vi "eodrecorder_looping_open.vi"() -> ()   [LabVIEW 2012]
uses:
  eodrecorderstates.ctl
  <vilib>/Utility/error.llb/DialogType.ctl
  <vilib>/_DAQmxBase/Internals/DAQmxBase Create Channel (AI-Voltage-Basic).vi
  <vilib>/_DAQmxBase/Internals/DAQmxBase Timing (Sample Clock).vi
  <vilib>/_DAQmxBase/Internals/DAQmxBase Read (Analog 2D DBL NChan NSamp).vi
panel:
  out "Recording Length (sec.)":dbl
  in  "Threshold":sgl
  in  "NumSamptoGrab":i32
  in  "SampleRate":dbl=10000.0
  in  "Channel":tag="Dev1/ai0"
  out "String":string
  out "Tab Control":enum32{"Live Data", "Edit Data", "View Data"}(tab)
  in  "Discard&Continue":bool
  in  "Save&Finish":bool
  in  "Save&Continue":bool
  in  "StartOver":bool
  in  "Tab Control 2":enum32{"Enter Data", "View Data"}(tab)
  out "Time":string
  out "Date":string
  in  "Specimen No.":string
  in  "Locality Code":string
  in  "Recording Temp ûC":string
  in  "Comments":string
  in  "Species":string
  in  "Gain":dbl(knob) scale=0.0..10.0
  in  "Coupling":bool
  in  "Wave Number":u16(slide) scale=0.0..1.0
  out "WaveformDisplay":T1(array[cluster])
  out "EodText":string[](array[string])
  out "Polarity":i32[](array[numeric])
  out "Npts":i32[](array[numeric])
  out "Srate":i32[](array[numeric])
  out "ADRange":dbl[](array[numeric])
  in  "WaveNumber":i32(slide) max=4 scale=0.0..1.0
  out "Waveform Graph":dbl[][](graph) caption="Measurement"
  in  "LiveDataMode":bool
  in  "Capture":bool
  in  "Stop":bool
  in  "Open Data":bool
  # "EOD Recorder v. 0.1a"
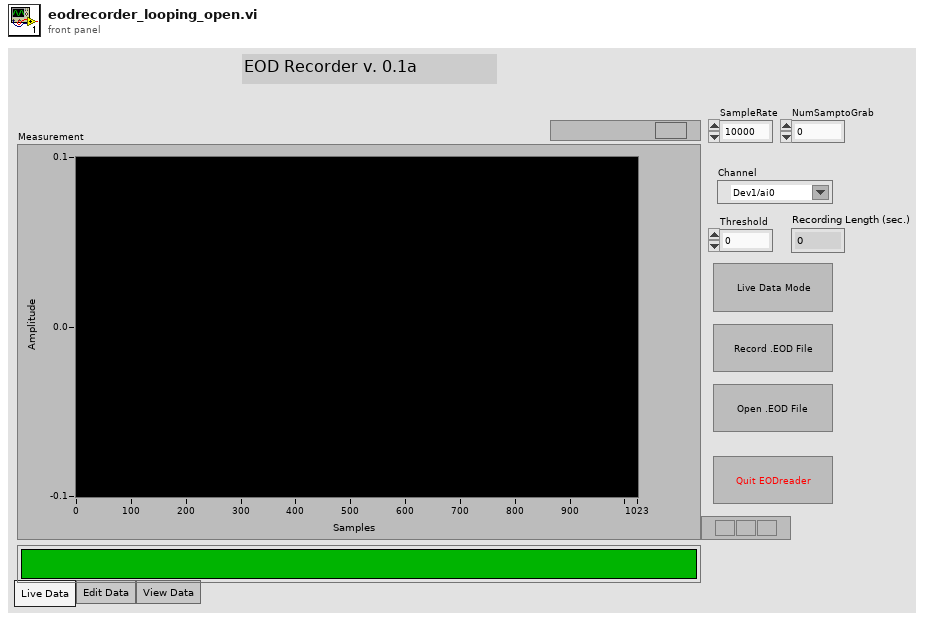
[diagram p1: front panel]
types:
  T1 = cluster{"Specimen No.":string, "Locality Code":string, "Species":string, "Recording Temp":string, "Comments 2":string, "Gain 2":dbl, "Coupling 2":bool, "Date 2":string, "Time 2":string}[]
  T2 = cluster{"data":dbl[][], "task ":refnum<k21>, "error ":errorcluster, "Min":dbl, "Max":dbl, "Srate":dbl, "WaveformData":cluster{"Nchar":i32[], "EodText":string[], "Nbits":i32[], "Nbytes":i32[], "userdata":dbl[][], "Polarity":i32[], "Srate":i32[], "ADRange":dbl[], "Npts":i32[], "Wave":dbl[][]}, "NumberofWavesLoaded":i32, "output array 2":cluster{"Specimen 2":string, "Location 2":string, "Species 2":string, "Temp 2":string, "Comments 2":string, "Gain 2":dbl, "Coupling 2":bool, "Date 2":string, "Time 2":string}[]}
  T3 = typedef "eodrecorderstates.ctl" = enum16{"stop", "initialize", "live data", "capture data", "analyze data", "open data", "display opened data", "write to file"}
  T4 = enum16{"Rising Edge", "Falling Edge", "Above Level", "Below Level", "When Inside Window", "When Outside Window"}
  T5 = enum16{"open", "replace", "create", "open or create", "replace or create", "replace or create with confirmation"}
  T6 = cluster{"Specimen 2":string, "Location 2":string, "Species 2":string, "Temp 2":string, "Comments 2":string, "Gain":dbl, "Coupling":bool, "Date 2":string, "Time 2":string}
  T7 = cluster{"Specimen 2":string, "Location 2":string, "Species 2":string, "Temp 2":string, "Comments 2":string, "Gain 2":dbl, "Coupling 2":bool, "Date 2":string, "Time 2":string}[]
  T8 = enum16{"big-endian, network order", "native, host order", "little-endian"}
  T9 = typedef "DialogType.ctl" = u16
  T10 = cluster{"Nchar":i32[], "EodText":string[], "Nbits":i32[], "Nbytes":i32[], "userdata":dbl[][], "Polarity":i32[], "Srate":i32[], "ADRange":dbl[], "Npts":i32[], "Wave":dbl[][]}
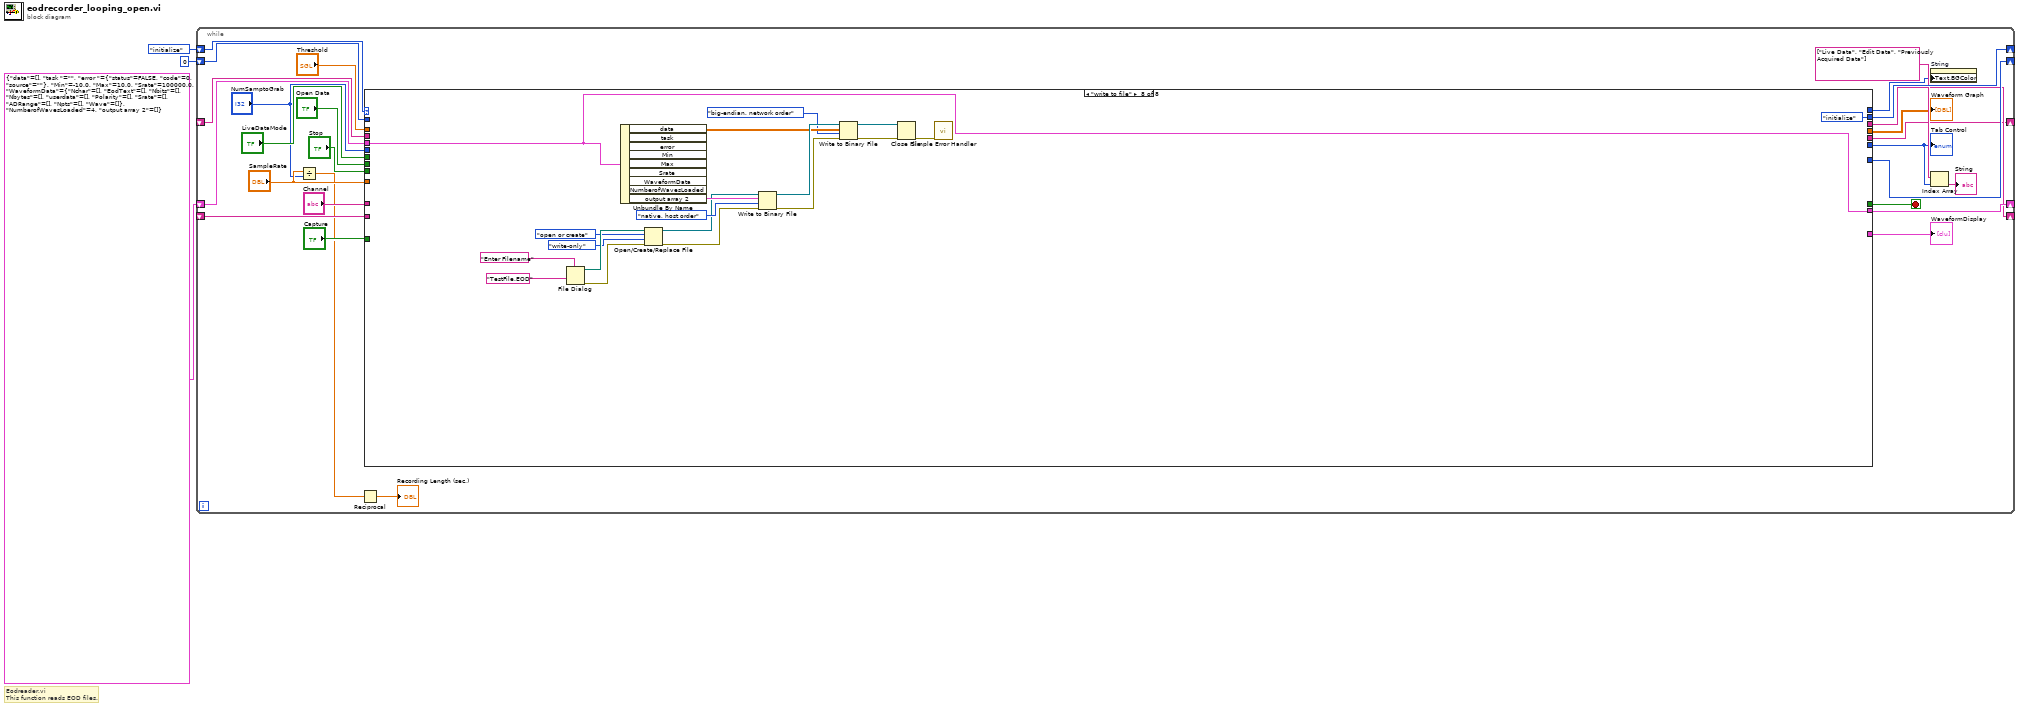
[diagram p0: block diagram]
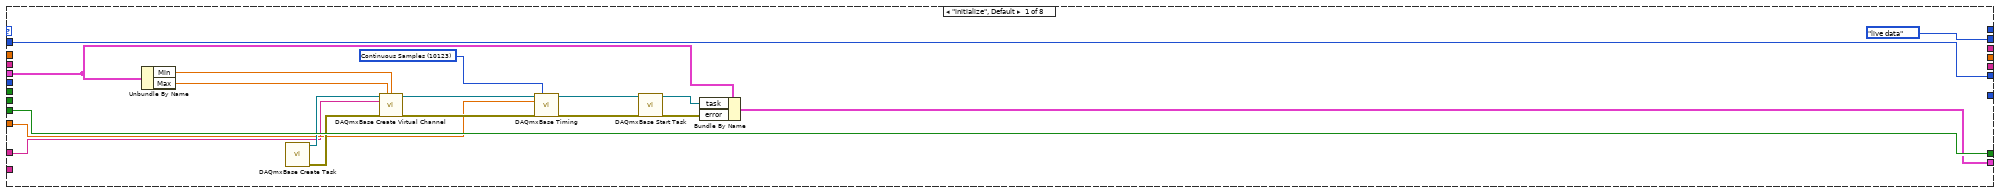
[diagram p2: hidden frame]
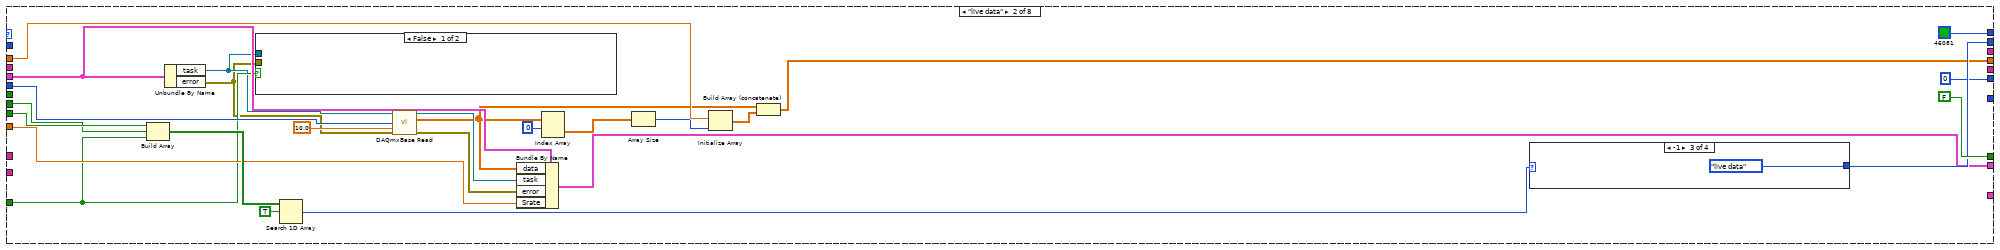
[diagram p3: hidden frame]
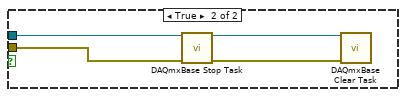
[diagram p4: hidden frame]
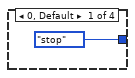
[diagram p5: hidden frame]
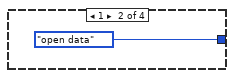
[diagram p6: hidden frame]
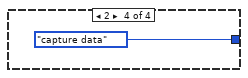
[diagram p7: hidden frame]
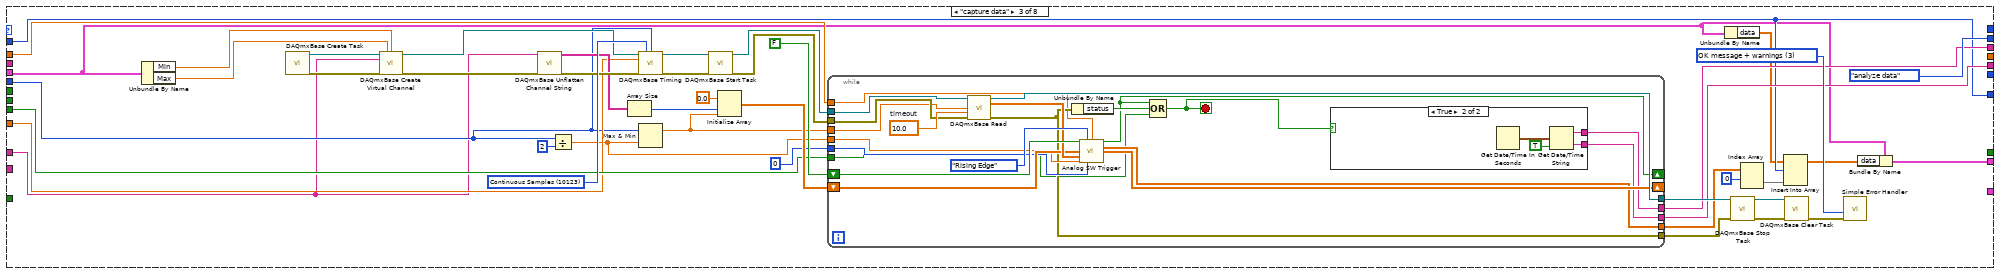
[diagram p8: hidden frame]
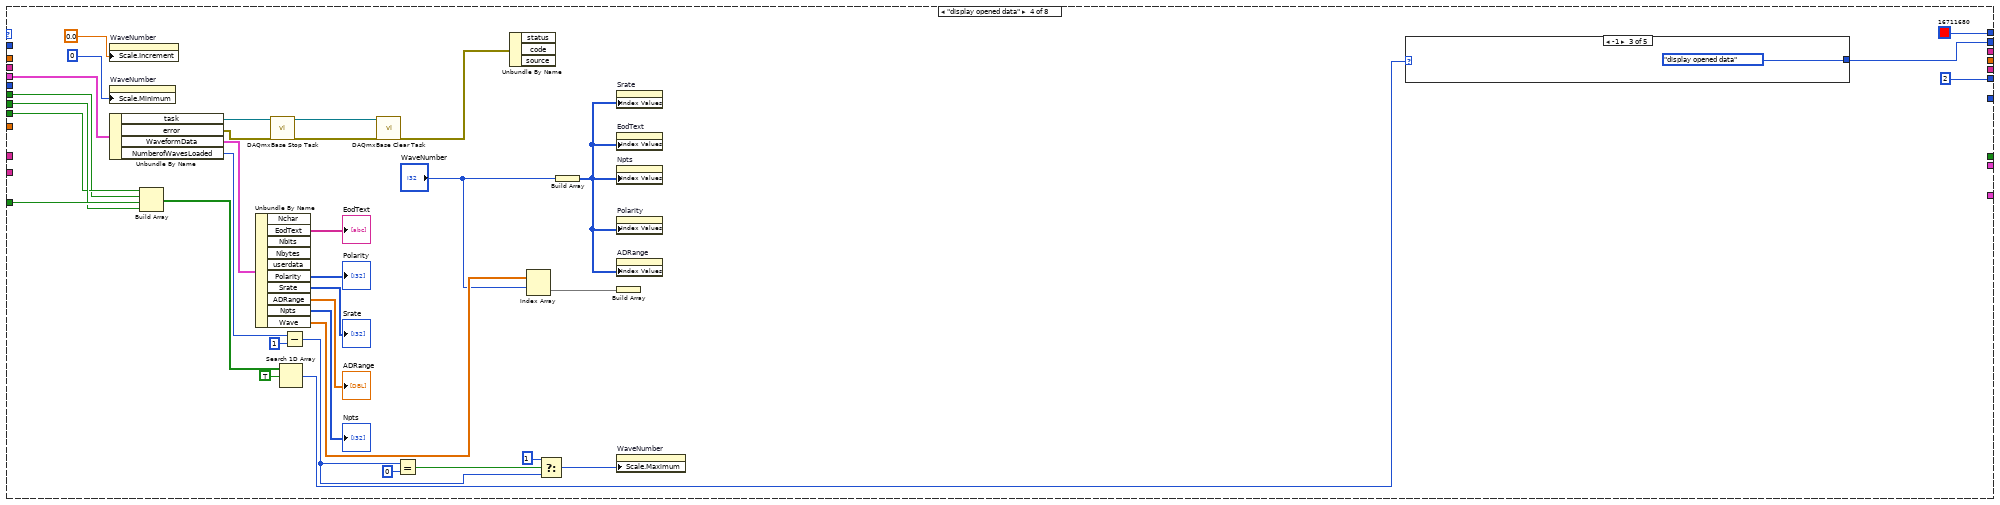
[diagram p10: hidden frame]
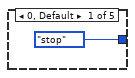
[diagram p11: hidden frame]
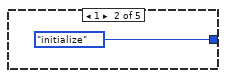
[diagram p12: hidden frame]
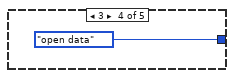
[diagram p13: hidden frame]
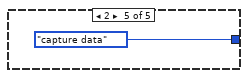
[diagram p14: hidden frame]
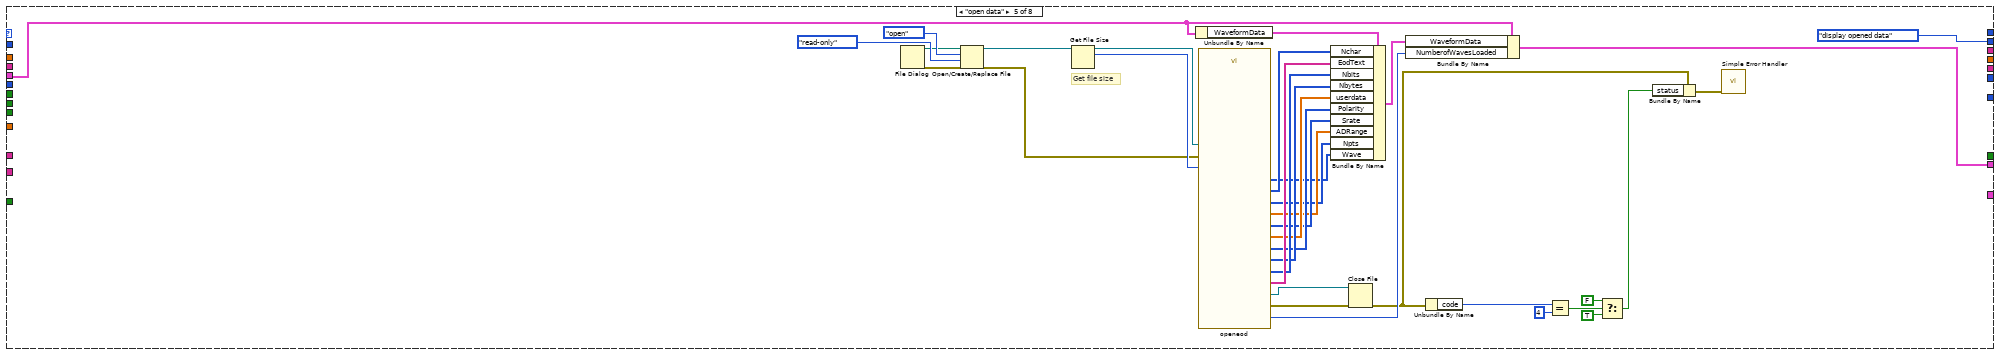
[diagram p15: hidden frame]
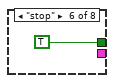
[diagram p16: hidden frame]
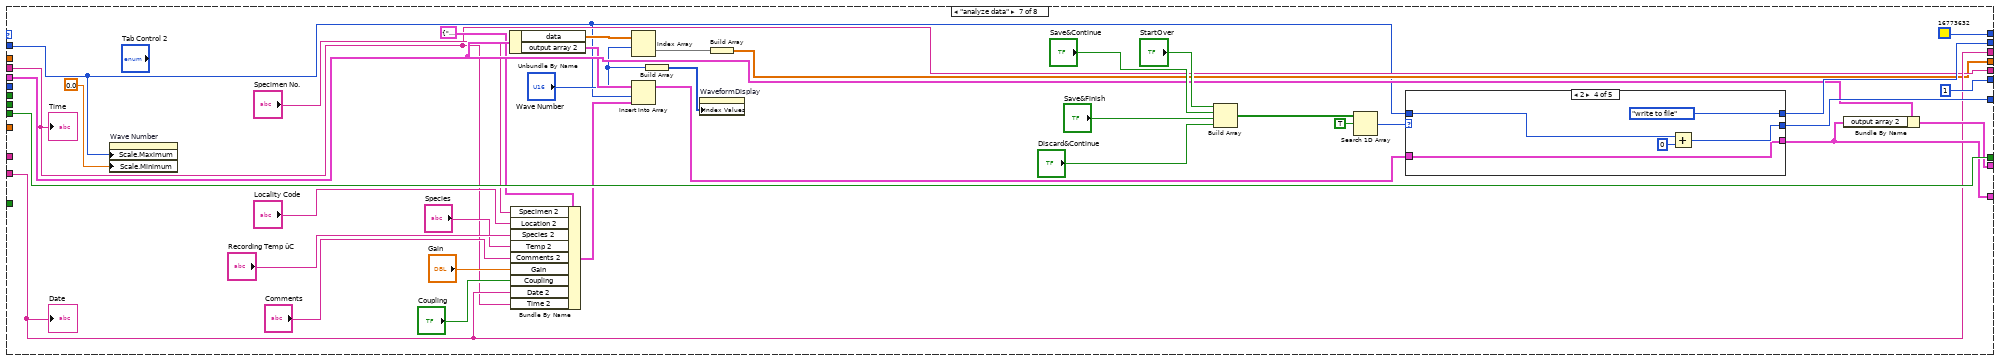
[diagram p17: hidden frame]
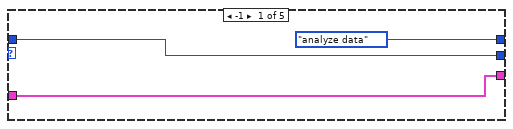
[diagram p18: hidden frame]
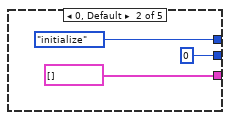
[diagram p19: hidden frame]
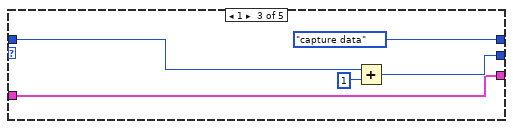
[diagram p20: hidden frame]
diagram:
  # "Eodreader.vi\nThis function reads EOD files."
  n1 = while {
    shift-right: [w29] -> _
    shift-left: eodrecorderstates."initialize" ("Enum") -> [w22]
    shift-right: [w15] -> _
    shift-left: T2 {"data"=[], "task "="", "error "={"status"=FALSE, "code"=0, "source"=""}, "Min"=-10.0, "Max"=10.0, "Srate"=100000.0, "WaveformData"={"Nchar"=[], "EodText"=[], "Nbits"=[], "Nbytes"=[], "userdata"=[], "Polarity"=[], "Srate"=[], "ADRange"=[], "Npts"=[], "Wave"=[]}, "NumberofWavesLoaded"=4, "output array 2"=[]} -> [w27]
    shift-right: [w16] -> _
    shift-left: u16 0 -> [w17]
    shift-right: [w12] -> _
    shift-left: _ -> [w10]
    shift-right: [w11] -> _
    shift-left: _ -> [w9]
    stop <- w30 stop-if-true
    n2 = Divide(x="SampleRate", y="NumSamptoGrab") -> (x/y=w5:dbl)
    n3 = Reciprocal(x=w5) -> (1/x=→"Recording Length (sec.)":dbl)
    n4 = case shown="\"write to file\"" w22 {
      tunnel: [w47 FALSE _ _ _ TRUE w257 _] -> w30
      tunnel: [eodrecorderstates."live data" ("Enum") w73 eodrecorderstates."analyze data" ("Enum") w185 eodrecorderstates."display opened data" ("Enum") _ w256 eodrecorderstates."initialize" ("Enum")] -> w29
      tunnel: "Stop" -> [w47 w72 w100 w179 _ _ w257 _]
      tunnel: w27 -> [w34 w68 w85 w151 w193 _ w247 w282]
      tunnel: "NumSamptoGrab" -> [_ w64 w97 _ _ _ _ _]
      tunnel: "SampleRate" -> [w35 w62 w98 _ _ _ _ _]
      tunnel: "Open Data" -> [_ w63 _ w181 _ _ _ _]
      tunnel: "Capture" -> [_ w60 _ w182 _ _ _ _]
      tunnel: "LiveDataMode" -> [_ _ _ w178 _ _ _ _]
      tunnel: "Threshold" -> [_ w61 w99 _ _ _ _ _]
      tunnel: [w33 0 _ 2 _ _ 1 _] -> w19
      tunnel: [_ u32 46081 _ u32 16711680 _ _ u32 16773632 _] -> w18
      tunnel: w17 -> [w33 _ w87 _ _ _ w226 _]
      tunnel: [_ _ w87 _ _ _ w255 _] -> w16
      tunnel: [w31 w50 w92 _ w191 _ w246 w282] -> w15
      tunnel: "Channel" -> [w32 _ w93 _ _ _ _ _]
      tunnel: [_ _ _ _ _ _ w244 _] -> w13
      tunnel: [_ _ w91 _ _ _ w234 _] -> w12
      tunnel: [_ _ w90 _ _ _ w233 _] -> w11
      tunnel: w10 -> [_ _ _ _ _ _ w234 _]
      tunnel: w9 -> [_ _ _ _ _ _ w233 _]
      tunnel: [_ w49 _ _ _ _ w228 _] -> w8
      frame "initialize", Default {
        w42 = 10123 items=["Finite Samples"=10178, "Continuous Samples"=10123] ("sample mode")
        n5 = Unbundle By Name(w34) -> ("Min"=w39:dbl, "Max"=w38:dbl)
        n6 = call <vilib>:"DAQmxBase Create Task.vi"() -> ("task out"=w45:refnum<k21>, "error out"=w46:errorcluster)  [unwired: 5 in, 9 out]
        n7 = call-poly <vilib>:"DAQmxBase Create Virtual Channel.vi"("task in"=w45, "maximum value"=w38, "minimum value"=w39, "physical channels"=w32, "error in"=w46) -> ("task out"=w43:refnum<k21>, "error out"=w44:errorcluster)  [unwired: 4 in, 5 out]
        n8 = call-poly <vilib>:"DAQmxBase Timing.vi"("task/channels in"=w43, "sample mode"=w42, "rate"=w35, "error in"=w44) -> ("task out"=w37:refnum<k21>, "error out"=w36:errorcluster)  [unwired: 3 in, 7 out]
        n9 = call <vilib>:"DAQmxBase Start Task.vi"("task/channels in"=w37, "error in"=w36) -> ("task out"=w41:refnum<k21>, "error out"=w40:errorcluster)  [unwired: 12 out]
        n10 = Bundle By Name(cluster=w34, "task"=w41, "error"=w40) -> (w31:T2)
      }
      frame "live data" {
        n11 = Build Array(w72, w63, w60) -> (w71:bool[])
        n12 = Unbundle By Name(w68) -> ("task"=w59:refnum<k21>, "error"=w58:errorcluster)
        n13 = case shown="False" w60 {
          tunnel: w59 -> [_ w78]
          tunnel: w58 -> [_ w77]
          frame False {
          }
          frame True {
            n14 = call <vilib>:"DAQmxBase Stop Task.vi"("task/channels in"=w78, "error in"=w77) -> ("task out"=w76:refnum<k21>, "error out"=w75:errorcluster)  [unwired: 12 in]
            n15 = call <vilib>:"DAQmxBase Clear Task.vi"("task in"=w76, "error in"=w75) -> ()  [unwired: 13 in, 1 out]
          }
        }
        n16 = Search 1D Array(1D array=w71, element=TRUE) -> (index of element=w69:i32)  [unwired: 1 in]
        n17 = call-poly <vilib>:"DAQmxBase Read.vi"("task/channels in"=w59, "number of samples per channel"=w64, "timeout"=10.0, "error in"=w58) -> ("task out"=w67:refnum<k21>, "data"=w53:dbl[][], "error out"=w66:errorcluster)  [unwired: 9 out]
        n18 = Bundle By Name(cluster=w68, "data"=w53, "task"=w67, "error"=w66, "Srate"=w62) -> (w50:T2)
        n19 = Index Array(array=w53, index (row)=0) -> (element=w55:dbl[])  [unwired: 1 in]
        n20 = Array Size(array=w55) -> (size(s)=w56:i32)
        n21 = Initialize Array(w61, w56) -> (w54:sgl[])
        n22 = Build Array (concatenate)(w53, w54) -> (w49:dbl[][])
        n23 = case shown="-1" w69 {
          tunnel: [eodrecorderstates."stop" ("Enum") eodrecorderstates."open data" ("Enum") eodrecorderstates."live data" ("Enum") eodrecorderstates."capture data" ("Enum")] -> w73
          frame 0, Default {
          }
          frame 1 {
          }
          frame -1 {
          }
          frame 2 {
          }
        }
      }
      frame "capture data" {
        w105 = T9 3 items=["no dialog", "OK message", "continue or stop message", "OK message + warnings", "continue/stop + warnings"] ("type of dialog (OK msg:1)")
        w125 = 10123 items=["Finite Samples"=10178, "Continuous Samples"=10123] ("sample mode")
        n24 = Unbundle By Name(w85) -> ("Min"=w122:dbl, "Max"=w121:dbl)
        n25 = call <vilib>:"DAQmxBase Create Task.vi"() -> ("task out"=w124:refnum<k21>, "error out"=w123:errorcluster)  [unwired: 14 in]
        n26 = call-poly <vilib>:"DAQmxBase Create Virtual Channel.vi"("task in"=w124, "maximum value"=w121, "minimum value"=w122, "physical channels"=w93, "error in"=w123) -> ("task out"=w120:refnum<k21>, "error out"=w117:errorcluster)  [unwired: 9 in]
        n27 = call "DAQmxBase Unflatten Channel String.vi"("names in"=w93, "error in"=w117) -> ("names out"=w115:string[], "error out"=w116:errorcluster)  [unwired: 12 in]
        n28 = Divide(x=w97, y=2) -> (x/y=w95:dbl)
        n29 = Array Size(array=w115) -> (size(s)=w114:i32)
        n30 = call-poly <vilib>:"DAQmxBase Timing.vi"("task/channels in"=w120, "sample mode"=w125, "samples per channel"=w97, "rate"=w98, "error in"=w116) -> ("task out"=w119:refnum<k21>, "error out"=w118:errorcluster)  [unwired: 2 in, 7 out]
        n31 = Max & Min(x=w97, y=w95) -> (max(x,y)=w107:dbl)  [unwired: 1 out]
        n32 = call <vilib>:"DAQmxBase Start Task.vi"("task/channels in"=w119, "error in"=w118) -> ("task out"=w111:refnum<k21>, "error out"=w112:errorcluster)  [unwired: 12 out]
        n33 = Initialize Array(0.0, w114, w107) -> (w110:dbl[][])
        n34 = while {
          tunnel: [w140] -> w102
          shift-right: [w139] -> _
          shift-left: FALSE ("Trigger Out") -> [w145]
          shift-right: [w133] -> _
          shift-left: w110 -> [w141]
          tunnel: w112 -> [w138]
          tunnel: w111 -> [w137]
          tunnel: w95 -> [w136]
          tunnel: 0 ("Channel Index") -> [w135]
          tunnel: w107 -> [w134]
          tunnel: [w132] -> w89
          tunnel: [w131] -> w101
          tunnel: w100 -> [w130]
          tunnel: w99 -> [w129]
          tunnel: [w127] -> w91
          tunnel: [w126] -> w90
          stop <- w128 stop-if-true
          w146 = 10.0  # timeout
          n35 = call-poly <vilib>:"DAQmxBase Read.vi"("task/channels in"=w137, "number of samples per channel"=w134, "timeout"=w146, "error in"=w138) -> ("task out"=w140:refnum<k21>, "data"=w142:dbl[][], "error out"=w131:errorcluster)  [unwired: 9 in]
          n36 = Unbundle By Name(w131) -> ("status"=w144:bool)
          n37 = call "Analog SW Trigger.vi"("Triggered?"=w145, "Condition"=T4."Rising Edge", "Level"=w129, "Initialized Data Array"=w141, "Input Raw Data"=w142, "Pretrigger Samples"=w136, "Index of Condition Channel"=w135) -> ("Trigger Out"=w139:bool, "Output Data (Scaled)"=w132:dbl[][], "Raw Data Out"=w133:dbl[][])  [unwired: 4 in, 2 out]
          n38 = Compound Arithmetic op=OR(w139, w144, w130) -> (w128:bool)
          n39 = case shown="True" w128 {
            tunnel: [_ w148] -> w127
            tunnel: [_ w147] -> w126
            frame False {
            }
            frame True {
              n40 = Get Date/Time In Seconds() -> (seconds since 1Jan1904=w150:timestamp)
              n41 = Get Date/Time String(seconds (now)=w150, want seconds? (F)=TRUE) -> (date string=w148:string, time string=w147:string)  [unwired: 1 in]
            }
          }
        }
        n42 = Unbundle By Name(w85) -> ("data"=w84:dbl[][])
        n43 = call <vilib>:"DAQmxBase Stop Task.vi"("task/channels in"=w102, "error in"=w101) -> ("task out"=w104:refnum<k21>, "error out"=w103:errorcluster)  [unwired: 12 in]
        n44 = Index Array(array=w89, index (row)=0) -> (element=w83:dbl[])  [unwired: 1 in]
        n45 = Insert Into Array(array=w84, index (row)=w87, new element=w83) -> (w86:dbl[][])  [unwired: 1 in]
        n46 = call <vilib>:"DAQmxBase Clear Task.vi"("task in"=w104, "error in"=w103) -> ("error out"=w106:errorcluster)  [unwired: 13 in]
        n47 = call <vilib>:"Simple Error Handler.vi"("type of dialog (OK msg:1)"=w105, "error in (no error)"=w106) -> ()  [unwired: 3 in, 5 out]
        n48 = Bundle By Name(cluster=w85, "data"=w86) -> (w92:T2)
      }
      frame "display opened data" {
        n49 = property on="WaveNumber" class="Slide (strict)"("Scale.Increment"=0.0 ("Scale.Range:Increment")) -> ()  [unwired: 2 in, 2 out]
        n50 = property on="WaveNumber" class="Slide (strict)"("Scale.Minimum"=0) -> ()  [unwired: 2 in, 2 out]
        n51 = Unbundle By Name(w151) -> ("task"=w174:refnum<k21>, "error"=w173:errorcluster, "WaveformData"=w172:T10, "NumberofWavesLoaded"=w160:i32)
        n52 = Build Array(w179, w178, w182, w181) -> (w184:bool[])
        n53 = Unbundle By Name(w172) -> ("EodText"=→"EodText":string[], "Polarity"=→"Polarity":i32[], "Srate"=→"Srate":i32[], "ADRange"=→"ADRange":dbl[], "Npts"=→"Npts":i32[], "Wave"=w164:dbl[][])  [unwired: 4 out]
        n54 = call <vilib>:"DAQmxBase Stop Task.vi"("task/channels in"=w174, "error in"=w173) -> ("task out"=w175:refnum<k21>, "error out"=w176:errorcluster)  [unwired: 12 in]
        n55 = Search 1D Array(1D array=w184, element=TRUE) -> (index of element=w180:i32)  [unwired: 1 in]
        n56 = Subtract(x=w160, y=1) -> (x-y=w155:i32)
        n57 = call <vilib>:"DAQmxBase Clear Task.vi"("task in"=w175, "error in"=w176) -> ("error out"=w177:errorcluster)  [unwired: 13 in]
        n58 = Equal?(x=w155, y=0) -> (x = y?=w156:bool)
        n59 = Unbundle By Name(w177) -> ()  [unwired: 3 out]
        n60 = Index Array(array=w164, index (row)="WaveNumber") -> (element=w162:dbl[])  [unwired: 1 in]
        n61 = Select(t=1, s=w156, f=w155) -> (s? t:f=w153:i32)
        n62 = Build Array("WaveNumber") -> (w166:i32[])
        n63 = property on="Srate" class="Arr (strict)"("Index Values"=w166) -> ()  [unwired: 2 in, 2 out]
        n64 = property on="EodText" class="Arr (strict)"("Index Values"=w166) -> ()  [unwired: 2 in, 2 out]
        n65 = property on="Npts" class="Arr (strict)"("Index Values"=w166) -> ()  [unwired: 2 in, 2 out]
        n66 = property on="Polarity" class="Arr (strict)"("Index Values"=w166) -> ()  [unwired: 2 in, 2 out]
        n67 = property on="ADRange" class="Arr (strict)"("Index Values"=w166) -> ()  [unwired: 2 in, 2 out]
        n68 = Build Array(w162) -> ()  [unwired: 1 out]
        n69 = property on="WaveNumber" class="Slide (strict)"("Scale.Maximum"=w153) -> ()  [unwired: 2 in, 2 out]
        n70 = case shown="-1" w180 {
          tunnel: [eodrecorderstates."stop" ("Enum") eodrecorderstates."initialize" ("Enum") eodrecorderstates."display opened data" ("Enum") eodrecorderstates."open data" ("Enum") eodrecorderstates."capture data" ("Enum")] -> w185
          frame 0, Default {
          }
          frame 1 {
          }
          frame -1 {
          }
          frame 3 {
          }
          frame 2 {
          }
        }
      }
      frame "open data" {
        # "Get file size"
        n71 = File Dialog() -> (0:w220:errorcluster, 3:w221:path)  [unwired: 7 in, 2 out]
        n72 = Open/Create/Replace File(file path (use dialog)=w221, error in=w220, operation (0:open)=T5."open", access (0:read/write)=enum16{"read/write", "read-only", "write-only"}."read-only") -> (refnum out=w209:refnum<file>, error out=w202:errorcluster)  [unwired: 2 in, 1 out]
        n73 = Get File Size(file=w209) -> (refnum out=w208:refnum<file>, size (in bytes)=w207:i64)  [unwired: 1 in, 1 out]
        n74 = Unbundle By Name(w193) -> ("WaveformData"=w219:T10)
        n75 = call "openeod.vi"("Byte Stream File in"=w208, "size (in bytes)"=w207, "error in (no error)"=w202) -> ("Wave"=w192:i16[][], "nchar"=w218:u8[], "polarity"=w214:i8[], "nWavepoints"=w210:u32[], "userdata"=w213:sgl[][], "Numeric"=w205:i32, "nbytes"=w215:i8[], "Byte Stream File out"=w204:refnum<file>, "ADrange"=w211:sgl[], "eodtext"=w217:string[], "srate"=w212:u32[], "nbits"=w216:i8[], "error out"=w203:errorcluster)  [unwired: 4 in]
        n76 = Bundle By Name(cluster=w219, "Nchar"=w218, "EodText"=w217, "Nbits"=w216, "Nbytes"=w215, "userdata"=w213, "Polarity"=w214, "Srate"=w212, "ADRange"=w211, "Npts"=w210, "Wave"=w192) -> (w206:T10)
        n77 = Close File(refnum=w204, error in=w203) -> (error out=w194:errorcluster)  [unwired: 1 out]
        n78 = Bundle By Name(cluster=w193, "WaveformData"=w206, "NumberofWavesLoaded"=w205) -> (w191:T2)
        n79 = Unbundle By Name(w194) -> ("code"=w201:i32)
        n80 = Equal?(x=w201, y=4) -> (x = y?=w199:bool)
        n81 = Select(t=FALSE, s=w199, f=TRUE) -> (s? t:f=w196:bool)
        n82 = Bundle By Name(cluster=w194, "status"=w196) -> (w195:errorcluster)
        n83 = call <vilib>:"Simple Error Handler.vi"("error in (no error)"=w195) -> ()  [unwired: 4 in, 5 out]
      }
      frame "stop" {
      }
      frame "analyze data" {
        n84 = property on="Wave Number" class="Slide (strict)"("Scale.Maximum"=w226, "Scale.Minimum"=0.0 ("Scale.Range:Minimum")) -> ()  [unwired: 2 in, 2 out]
        n85 = Unbundle By Name(w247) -> ("data"=w232:dbl[][], "output array 2"=w245:T7)
        n86 = Bundle By Name(cluster=T6 {"Specimen 2"="", "Location 2"="", "Species 2"="", "Temp 2"="", "Comments 2"="", "Gain"=50.0, "Coupling"=TRUE, "Date 2"="", "Time 2"=""} ("WaveformDescribe 2"), "Specimen 2"="Specimen No.", "Location 2"="Locality Code", "Species 2"="Species", "Temp 2"="Recording Temp ûC", "Comments 2"="Comments", "Gain"="Gain", "Coupling"="Coupling", "Date 2"=w234, "Time 2"=w233) -> (w235:T6)
        n87 = Index Array(array=w232, index (row)="Wave Number") -> (element=w229:dbl[])  [unwired: 1 in]
        n88 = Insert Into Array(array=w245, index=w226, new element=w235) -> (w249:T7)
        n89 = Build Array("Wave Number") -> (w231:u16[])
        n90 = property on="WaveformDisplay" class="Arr (strict)"("Index Values"=w231) -> ()  [unwired: 2 in, 2 out]
        n91 = Build Array(w229) -> (w228:dbl[][])
        n92 = Build Array("StartOver", "Save&Continue", "Save&Finish", "Discard&Continue") -> (w258:bool[])
        n93 = Search 1D Array(1D array=w258, element=TRUE) -> (index of element=w250:i32)  [unwired: 1 in]
        n94 = case shown="2" w250 {
          tunnel: [w262 0 w270 w275 w280] -> w255
          tunnel: w226 -> [w262 _ w269 w274 w279]
          tunnel: [eodrecorderstates."analyze data" ("Enum") eodrecorderstates."initialize" ("Enum") eodrecorderstates."capture data" ("Enum") eodrecorderstates."write to file" ("Enum") eodrecorderstates."capture data" ("Enum")] -> w256
          tunnel: [w261 T7 [] ("output array 2") w267 w272 w277] -> w244
          tunnel: w249 -> [w261 _ w267 w272 w277]
          frame -1 {
          }
          frame 0, Default {
          }
          frame 1 {
            n95 = Add(x=w269, y=1) -> (x+y=w270:i32)
          }
          frame 2 {
            n96 = Add(x=w274, y=0) -> (x+y=w275:i32)
          }
          frame 3 {
            n97 = Add(x=w279, y=0) -> (x+y=w280:i32)
          }
        }
        n98 = Bundle By Name(cluster=w247, "output array 2"=w244) -> (w246:T2)
        "Time" <- w233
        "Date" <- w234
      }
      frame "write to file" {
        n99 = File Dialog(7:"Enter Filename" ("prompt"), 9:"TestFile.EOD" ("default name")) -> (0:w292:errorcluster, 3:w298:path)  [unwired: 5 in, 2 out]
        n100 = Unbundle By Name(w282) -> ("data"=w285:dbl[][], "output array 2"=w300:T7)  [unwired: 7 out]
        n101 = Open/Create/Replace File(file path (use dialog)=w298, error in=w292, operation (0:open)=T5."open or create", access (0:read/write)=enum16{"read/write", "read-only", "write-only"}."write-only") -> (refnum out=w294:refnum<file>, error out=w293:errorcluster)  [unwired: 2 in, 1 out]
        n102 = Write to Binary File(file (use dialog)=w294, data=w300, error in=w293, 9:T8."native, host order" ("byte order (0:big-endian, network order)")) -> (refnum out=w289:refnum<file>, error out=w288:errorcluster)  [unwired: 2 in, 1 out]
        n103 = Write to Binary File(file (use dialog)=w289, data=w285, error in=w288, 9:T8."big-endian, network order" ("byte order (0:big-endian, network order)")) -> (refnum out=w286:refnum<file>, error out=w287:errorcluster)  [unwired: 2 in, 1 out]
        n104 = Close File(refnum=w286, error in=w287) -> (error out=w291:errorcluster)  [unwired: 1 out]
        n105 = call <vilib>:"Simple Error Handler.vi"("error in (no error)"=w291) -> ()  [unwired: 4 in, 5 out]
      }
    }
    "Waveform Graph" <- w8
    "Tab Control" <- w19
    "WaveformDisplay" <- w13
    n106 = property on="String" class="Str"("Text.BGColor"=w18) -> ()  [unwired: 2 in, 2 out]
    n107 = Index Array(array=string[] ["Live Data", "Edit Data", "Previously Acquired Data"], index=w19) -> (element=→"String":string)
  }
